vi "Save Options Selection (SubVI).vi"(11 "Options Selection":i32[](array[numeric])) -> ()   [LabVIEW 2020]
uses:
  <vilib>/Utility/config.llb/Write Key (I32).vi
  <vilib>/Utility/config.llb/NI_LVConfig.lvlib
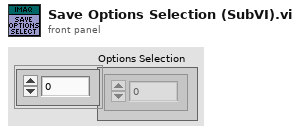
[diagram p1: front panel]
types:
  T1 = typedef "NI_LVConfig.lvlib/Config Data RefNum.ctl" = refnum<k1>
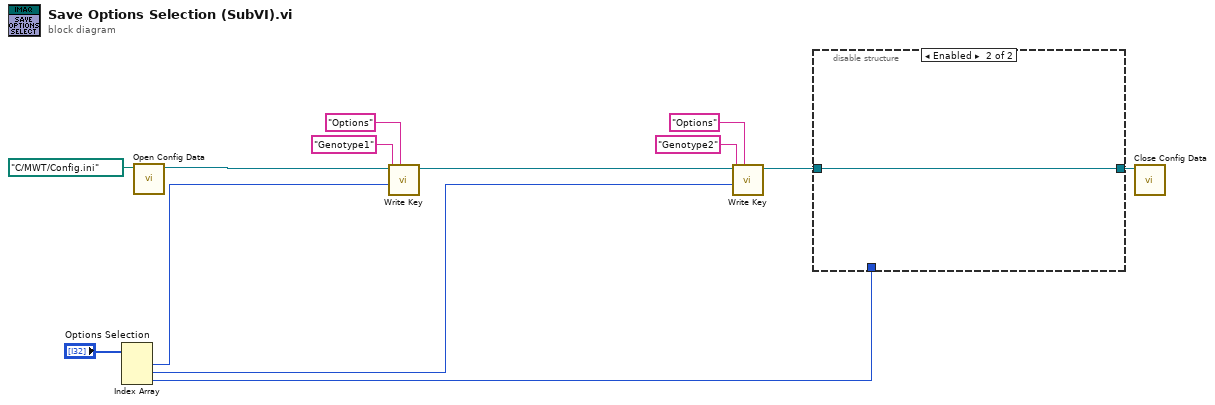
[diagram p0: block diagram]
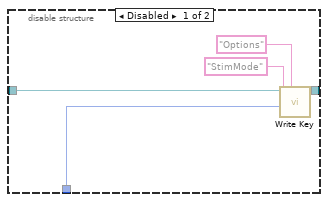
[diagram p2: hidden frame]
diagram:
  n1 = Index Array(array="Options Selection") -> (element #1=w7:i32, element #2=w6:i32, element #3=w5:i32)  [unwired: 3 in]
  n2 = call <vilib>:"Open Config Data.vi"("configuration file path"=path "C:/MWT/Config.ini") -> ("refnum"=w13:T1)  [unwired: 8 in, 2 out]
  n3 = call-poly <vilib>:"Write Key.vi"("section"="Options", "value"=w7, "key"="Genotype1" ("section"), "refnum"=w13) -> ("refnum out"=w11:T1)  [unwired: 5 in, 2 out]
  n4 = call-poly <vilib>:"Write Key.vi"("section"="Options", "value"=w6, "key"="Genotype2" ("section"), "refnum"=w11) -> ("refnum out"=w10:T1)  [unwired: 5 in, 2 out]
  n5 = disable-structure shown="Enabled" {
    disable-tunnel: w10 -> [w18 w19]
    disable-tunnel: [w17 w19] -> w9
    disable-tunnel: w5 -> [w16 _]
    frame Disabled {
      n6 = call-poly <vilib>:"Write Key.vi"("section"="Options", "value"=w16, "key"="StimMode" ("section"), "refnum"=w18) -> ("refnum out"=w17:T1)  [unwired: 5 in, 2 out]
    }
    frame Enabled {
    }
  }
  n7 = call <vilib>:"Close Config Data.vi"("refnum"=w9) -> ()  [unwired: 9 in, 2 out]
